vi "S2C_IMAGE_Proc_Acknowledge.vi"(8 "Error In":errorcluster, 11 "ImagePath":path) -> (0 "Error Out":errorcluster)   [LabVIEW 2015]
panel:
  in  "Ack":bool
  out "Image":picture
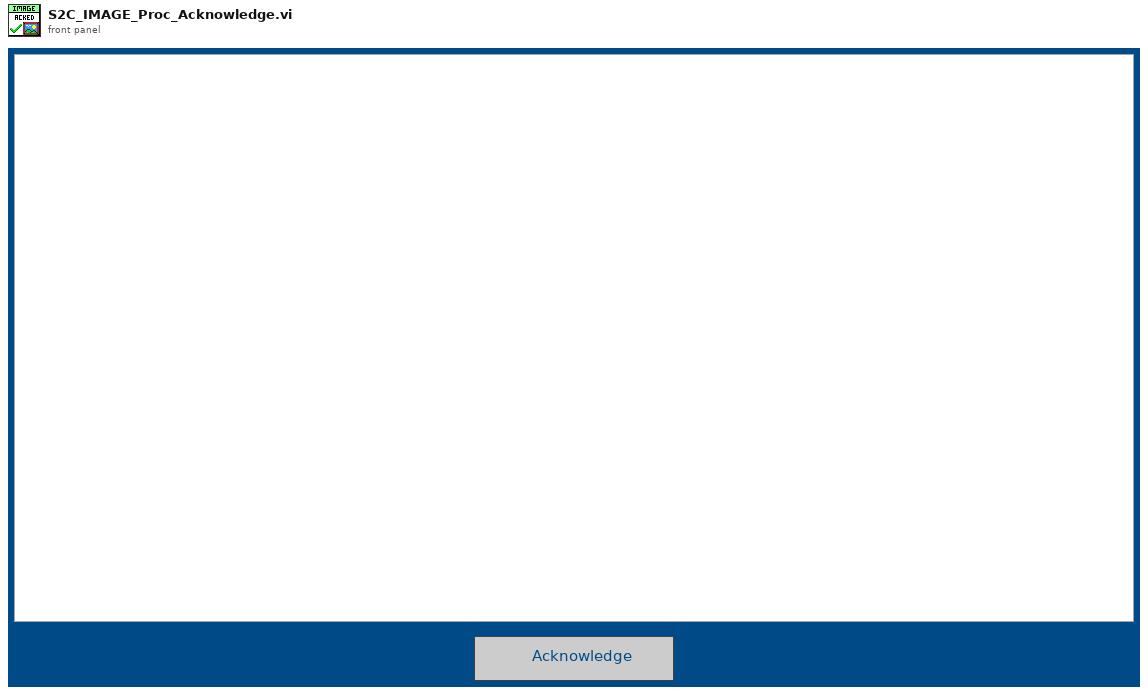
[diagram p1: front panel]
types:
  T1 = cluster{"Left":i16, "Top":i16, "Right":i16, "Bottom":i16}
  T2 = enum32{"Invalid", "Standard", "Closed", "Hidden", "Minimized", "Maximized"}
  T3 = typedef "imagedata.ctl" = cluster{"image type":i32, "image depth":i32, "image":u8[], "mask":u8[], "colors":u32[], "Rectangle":cluster{"left":i16, "top":i16, "right":i16, "bottom":i16}}
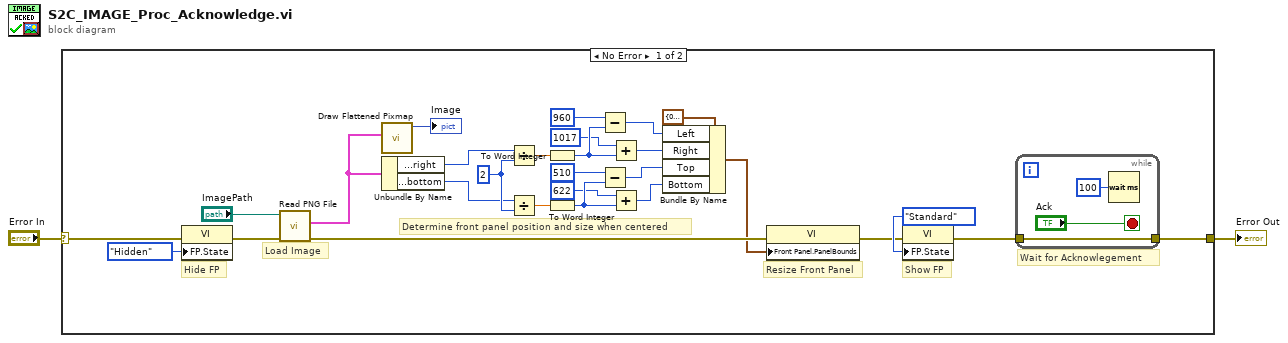
[diagram p0: block diagram]
diagram:
  n1 = case shown="No Error" "Error In" {
    selector: "Error In" -> [w26 w34]
    tunnel: [w28 w34] -> w1
    frame No Error {
      w20 = i16 2 ("y")
      # "Show FP"
      # "Resize Front Panel"
      # "Determine front panel position and size when centered"
      # "Hide FP"
      # "Wait for Acknowlegement"
      # "Load Image"
      n2 = property class="VI"(error in=w26, "FP.State"=T2."Hidden" ("Front Panel Window:State")) -> (error out=w24:errorcluster)  [unwired: 1 in, 1 out]
      n3 = call <vilib>:"Read PNG File.vi"("error in (no error)"=w24, "path to PNG file"="ImagePath") -> ("error out"=w7:errorcluster, "image data"=w27:T3)  [unwired: 7 in, 1 out]
      n4 = call <vilib>:"Draw Flattened Pixmap.vi"("image data"=w27) -> ("new picture"=→"Image":picture)  [unwired: 8 in]
      n5 = Unbundle By Name(w27) -> ("Rectangle.right"=w17:i16, "Rectangle.bottom"=w19:i16)
      n6 = Divide(x=w17, y=w20) -> (x/y=w18:dbl)
      n7 = Divide(x=w19, y=w20) -> (x/y=w12:dbl)
      n8 = To Word Integer(number=w18) -> (16bit integer=w15:i16)
      n9 = To Word Integer(number=w12) -> (16bit integer=w14:i16)
      n10 = Subtract(x=i16 960, y=w15) -> (x-y=w11:i16)
      n11 = Subtract(x=i16 510, y=w14) -> (x-y=w9:i16)
      n12 = Add(x=i16 1017, y=w15) -> (x+y=w10:i16)
      n13 = Add(x=i16 622, y=w14) -> (x+y=w8:i16)
      n14 = Bundle By Name(cluster=T1 {"Left"=0, "Top"=0, "Right"=0, "Bottom"=0} ("Front Panel Window:Panel Bounds"), "Left"=w11, "Right"=w10, "Top"=w9, "Bottom"=w8) -> (w6:T1)
      n15 = property class="VI"(error in=w7, "Front Panel.PanelBounds"=w6) -> (error out=w22:errorcluster)  [unwired: 1 in, 1 out]
      n16 = property class="VI"(error in=w22, "FP.State"=T2."Standard" ("Front Panel Window:State")) -> (error out=w21:errorcluster)  [unwired: 1 in, 1 out]
      n17 = while {
        tunnel: w21 -> [w33]
        tunnel: [w33] -> w28
        stop <- "Ack" stop-if-true
        n18 = Wait (ms)(milliseconds to wait=u32 100) -> ()  [unwired: 1 out]
      }
    }
    frame Error {
    }
  }
  "Error Out" <- w1
